vi "Arm.vi"(4 "AllUp":bool, 5 "MostUp":bool, 6 "MostDown":bool, 7 "AllDown":bool) -> ()   [LabVIEW 2017]
uses:
  <vilib>/Rock Robotics/WPI/Solenoid/Deprecated/WPI_SolenoidSetBool.vi
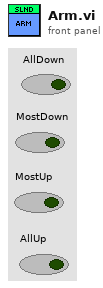
[diagram p1: front panel]
types:
  T1 = typedef "WPI_SolenoidDevRef.ctl" = cluster{"DevStatus":errorcluster, "Pneumatics Control Module":u8, "Forward Solenoid Channel":T2, "Reverse Solenoid Channel":T2}
  T2 = typedef "WPI_SolenoidChannel.ctl" = enum8{"Solenoid 0", "Solenoid 1", "Solenoid 2", "Solenoid 3", "Solenoid 4", "Solenoid 5", "Solenoid 6", "Solenoid 7", "Invalid"}
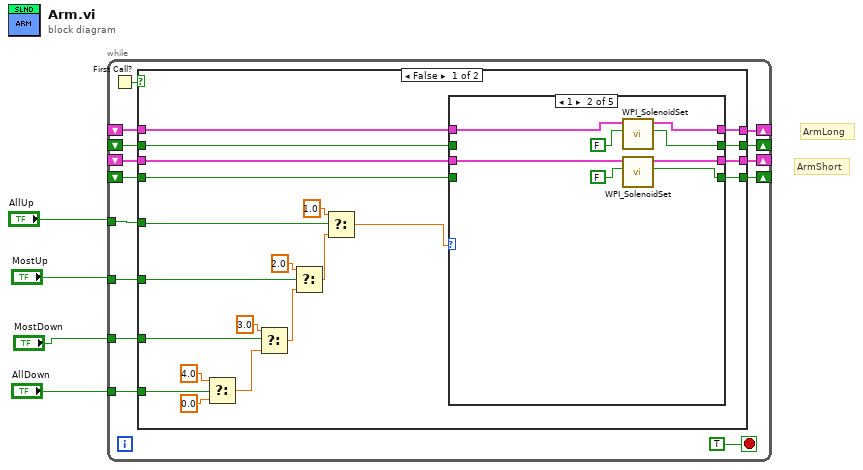
[diagram p0: block diagram]
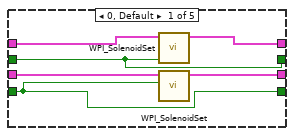
[diagram p2: hidden frame]
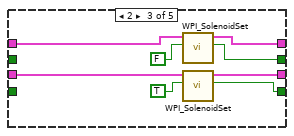
[diagram p3: hidden frame]
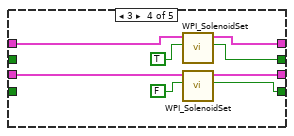
[diagram p4: hidden frame]
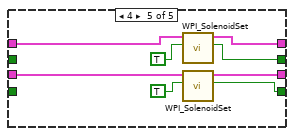
[diagram p5: hidden frame]
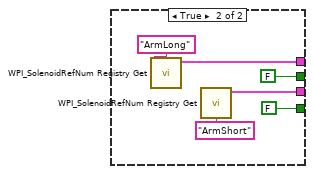
[diagram p6: hidden frame]
diagram:
  # "ArmShort"
  # "ArmLong"
  n1 = while {
    shift-right: [w16] -> _
    shift-left: _ -> [w15]
    tunnel: "AllUp" -> [w14]
    shift-right: [w13] -> _
    shift-left: _ -> [w12]
    shift-right: [w11] -> _
    shift-left: _ -> [w5]
    shift-right: [w10] -> _
    shift-left: _ -> [w9]
    tunnel: "MostUp" -> [w8]
    tunnel: "MostDown" -> [w7]
    tunnel: "AllDown" -> [w6]
    stop <- TRUE stop-if-true
    n2 = First Call?() -> (First Call?: T/F=w17:bool)
    n3 = case shown="False" w17 {
      tunnel: [w29 w74] -> w16
      tunnel: w15 -> [w30 _]
      tunnel: w14 -> [w38 _]
      tunnel: [w27 FALSE] -> w13
      tunnel: w12 -> [w28 _]
      tunnel: [w25 w71] -> w11
      tunnel: [w23 FALSE] -> w10
      tunnel: w9 -> [w24 _]
      tunnel: w8 -> [w36 _]
      tunnel: w7 -> [w34 _]
      tunnel: w6 -> [w31 _]
      tunnel: w5 -> [w26 _]
      frame False {
        n4 = Select(t=4.0, s=w31, f=0.0 ("t")) -> (s? t:f=w22:dbl)
        n5 = Select(t=3.0, s=w34, f=w22) -> (s? t:f=w21:dbl)
        n6 = Select(t=2.0, s=w36, f=w21) -> (s? t:f=w20:dbl)
        n7 = Select(t=1.0, s=w38, f=w20) -> (s? t:f=w19:dbl)
        n8 = case shown="1" w19 {
          tunnel: w30 -> [w43 w51 w57 w63 w69]
          tunnel: [w45 w50 w56 w62 w68] -> w29
          tunnel: w28 -> [w41 _ _ _ _]
          tunnel: [w41 w47 w53 w59 w65] -> w27
          tunnel: w26 -> [w42 w49 w55 w61 w67]
          tunnel: [w44 w48 w54 w60 w66] -> w25
          tunnel: w24 -> [w40 _ _ _ _]
          tunnel: [w40 w46 w52 w58 w64] -> w23
          frame 0, Default {
            n9 = call-poly <vilib>:"WPI_SolenoidSet.vi"("Value"=w41, "SolenoidDevRef"=w43) -> ("SolenoidDevRef"=w45:T1)  [unwired: 8 in, 1 out]
            n10 = call-poly <vilib>:"WPI_SolenoidSet.vi"("Value"=w40, "SolenoidDevRef"=w42) -> ("SolenoidDevRef"=w44:T1)  [unwired: 8 in, 1 out]
          }
          frame 1 {
            w46 = FALSE
            w47 = FALSE
            n11 = call-poly <vilib>:"WPI_SolenoidSet.vi"("Value"=w47, "SolenoidDevRef"=w51) -> ("SolenoidDevRef"=w50:T1)  [unwired: 8 in, 1 out]
            n12 = call-poly <vilib>:"WPI_SolenoidSet.vi"("Value"=w46, "SolenoidDevRef"=w49) -> ("SolenoidDevRef"=w48:T1)  [unwired: 8 in, 1 out]
          }
          frame 2 {
            w52 = TRUE
            w53 = FALSE
            n13 = call-poly <vilib>:"WPI_SolenoidSet.vi"("Value"=w53, "SolenoidDevRef"=w57) -> ("SolenoidDevRef"=w56:T1)  [unwired: 8 in, 1 out]
            n14 = call-poly <vilib>:"WPI_SolenoidSet.vi"("Value"=w52, "SolenoidDevRef"=w55) -> ("SolenoidDevRef"=w54:T1)  [unwired: 8 in, 1 out]
          }
          frame 3 {
            w58 = FALSE
            w59 = TRUE
            n15 = call-poly <vilib>:"WPI_SolenoidSet.vi"("Value"=w59, "SolenoidDevRef"=w63) -> ("SolenoidDevRef"=w62:T1)  [unwired: 8 in, 1 out]
            n16 = call-poly <vilib>:"WPI_SolenoidSet.vi"("Value"=w58, "SolenoidDevRef"=w61) -> ("SolenoidDevRef"=w60:T1)  [unwired: 8 in, 1 out]
          }
          frame 4 {
            w64 = TRUE
            w65 = TRUE
            n17 = call-poly <vilib>:"WPI_SolenoidSet.vi"("Value"=w65, "SolenoidDevRef"=w69) -> ("SolenoidDevRef"=w68:T1)  [unwired: 8 in, 1 out]
            n18 = call-poly <vilib>:"WPI_SolenoidSet.vi"("Value"=w64, "SolenoidDevRef"=w67) -> ("SolenoidDevRef"=w66:T1)  [unwired: 8 in, 1 out]
          }
        }
      }
      frame True {
        n19 = call <vilib>:"WPI_SolenoidRefNum Registry Get.vi"("refnum name"="ArmLong") -> ("SolenoidDevRef"=w74:T1)  [unwired: 9 in, 1 out]
        n20 = call <vilib>:"WPI_SolenoidRefNum Registry Get.vi"("refnum name"="ArmShort") -> ("SolenoidDevRef"=w71:T1)  [unwired: 9 in, 1 out]
      }
    }
  }
